vi "ABB Default VT-CT Ratios.vi"() -> ()   [LabVIEW 2017]
uses:
  ABB global.vi
panel:
  in  "exit":bool
  in  "Default VT and CT Ratios":T1
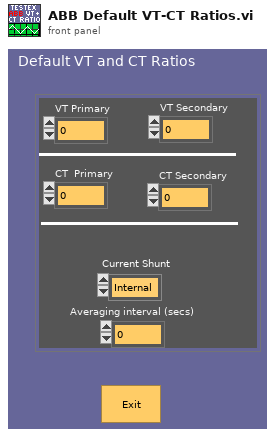
[diagram p1: front panel]
types:
  T1 = cluster{"VT Primary":dbl, "VT Secondary":dbl, "CT  Primary":dbl, "CT Secondary":dbl, "Current Shunt":enum16{"Internal", "External"}, "Averaging interval (secs)":dbl}
  T2 = cluster{"VT Primary":dbl, "VT Secondary":dbl, "CT  Primary":dbl, "CT Secondary":dbl, "Current Shunt":enum16{"Internal", "External"}, "Averaging interval":dbl}
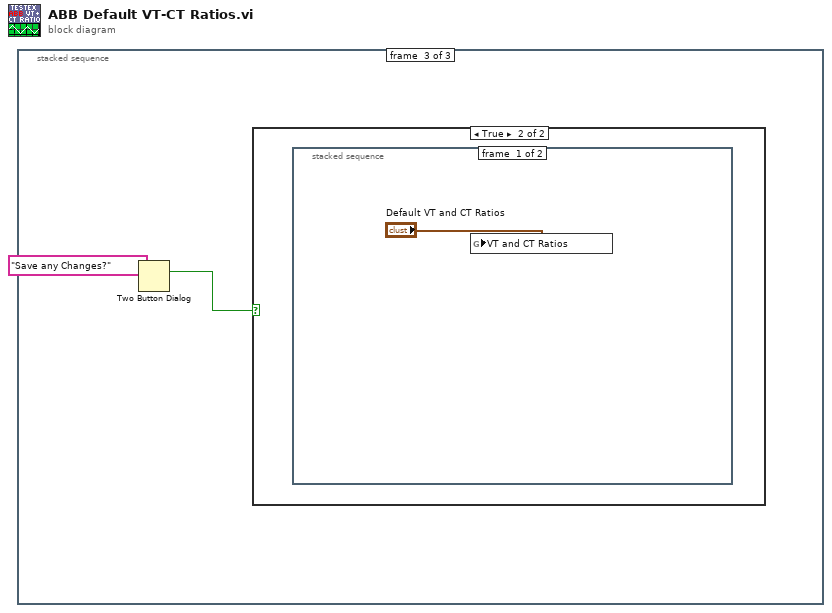
[diagram p0: block diagram]
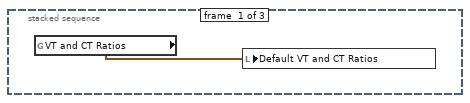
[diagram p2: hidden frame]
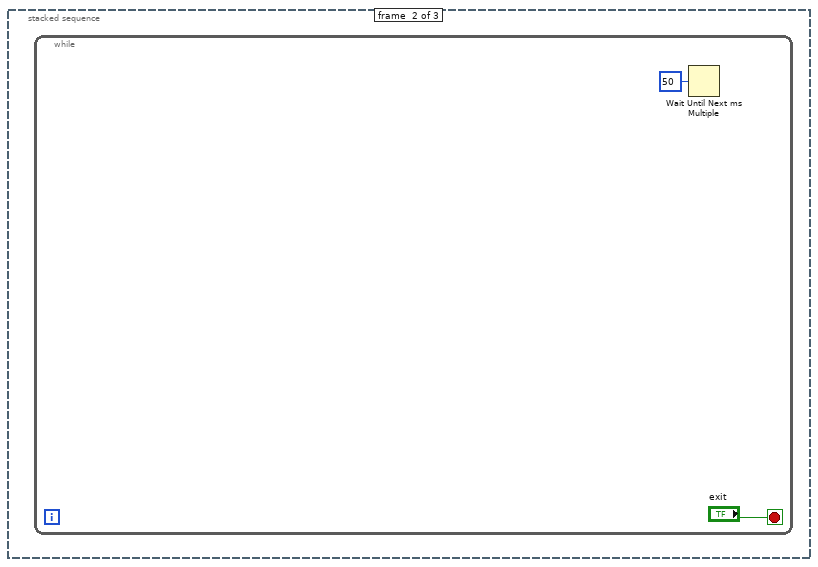
[diagram p3: hidden frame]
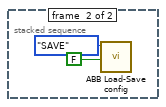
[diagram p5: hidden frame]
diagram:
  n1 = stacked-sequence {
    frame #0 {
      n2 = global read "ABB global.vi" "VT and CT Ratios"() -> (w1:T2)
      n3 = local write "Default VT and CT Ratios"(w1) -> ()
    }
    frame #1 {
      n4 = while {
        stop <- "exit" stop-if-true
        n5 = Wait Until Next ms Multiple(millisecond multiple=u32 50) -> ()  [unwired: 1 out]
      }
    }
    frame #2 {
      n6 = Two Button Dialog(message="Save any Changes?") -> (T button?=w5:bool)  [unwired: 2 in]
      n7 = case shown="True" w5 {
        frame False {
        }
        frame True {
          n8 = stacked-sequence {
            frame #0 {
              n9 = global write "ABB global.vi" "VT and CT Ratios"("Default VT and CT Ratios") -> ()
            }
            frame #1 {
              n10 = call "ABB Load-Save config.vi"("confirm save"=FALSE, "Mode"=enum16{"LOAD", "SAVE"}."SAVE") -> ()  [unwired: 10 in]
            }
          }
        }
      }
    }
  }
